vi "Format Basic String.vi"(10 "String":string) -> (2 "Formatted Basic String":string)   [LabVIEW 2019, in "BlueTOMLSerializer.lvlib"]
uses:
  BlueTOMLSerializer.lvlib
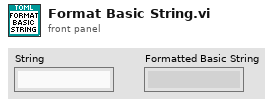
[diagram p1: front panel]
types:
  T1 = cluster{"replace string (\"\")":string, "replace string (\"\") 2":string}[]
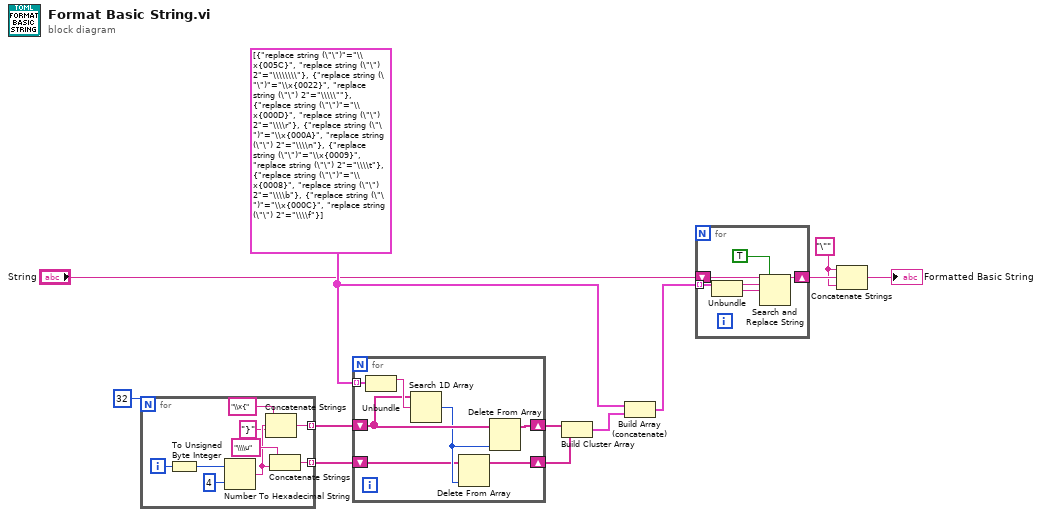
[diagram p0: block diagram]
diagram:
  w11 = "\"" ("string")
  w8 = T1 [{"replace string (\"\")"="\\x{005C}", "replace string (\"\") 2"="\\\\\\\\"}, {"replace string (\"\")"="\\x{0022}", "replace string (\"\") 2"="\\\\\""}, {"replace string (\"\")"="\\x{000D}", "replace string (\"\") 2"="\\\\r"}, {"replace string (\"\")"="\\x{000A}", "replace string (\"\") 2"="\\\\n"}, {"replace string (\"\")"="\\x{0009}", "replace string (\"\") 2"="\\\\t"}, {"replace string (\"\")"="\\x{0008}", "replace string (\"\") 2"="\\\\b"}, {"replace string (\"\")"="\\x{000C}", "replace string (\"\") 2"="\\\\f"}]
  n1 = for {
    N: 32 -> [_]
    tunnel: [w18] -> w5 mode=indexing
    tunnel: [w13] -> w4 mode=indexing
    i -> [w21]
    n2 = To Unsigned Byte Integer(number=w21) -> (unsigned 8bit integer=w16:u8)
    n3 = Number To Hexadecimal String(1:i16 4 ("width (-)"), 2:w16) -> (0:w15:string)
    n4 = Concatenate Strings("\\x{" ("string"), w15, "}" ("string")) -> (w13:string)
    n5 = Concatenate Strings("\\\\u" ("string"), w15) -> (w18:string)
  }
  n6 = for {
    tunnel: w8 -> [w28] mode=indexing
    shift-right: [w26] -> w6
    shift-left: w4 -> [w25]
    shift-right: [w23] -> w3
    shift-left: w5 -> [w22]
    n7 = Unbundle(w28) -> ("replace string (\"\")"=w27:string)  [unwired: 1 out]
    n8 = Search 1D Array(1D array=w25, element=w27) -> (index of element=w24:i32)  [unwired: 1 in]
    n9 = Delete From Array(array=w22, index=w24) -> (array with subset deleted=w23:string[])  [unwired: 1 in, 1 out]
    n10 = Delete From Array(array=w25, index=w24) -> (array with subset deleted=w26:string[])  [unwired: 1 in, 1 out]
  }
  n11 = Build Cluster Array(w6, w3) -> (w9:cluster{string, string}[])
  n12 = Build Array (concatenate)(w8, w9) -> (w7:T1)
  n13 = for {
    tunnel: w7 -> [w32] mode=indexing
    shift-right: [w29] -> w12
    shift-left: "String" -> [w34]
    n14 = Unbundle(w32) -> ("replace string (\"\")"=w31:string, "replace string (\"\") 2"=w30:string)
    n15 = Search and Replace String(replace all?=TRUE ("replace all? (F)"), input string=w34, search string=w31, replace string=w30) -> (result string=w29:string)  [unwired: 4 in, 3 out]
  }
  n16 = Concatenate Strings(w11, w12, w11) -> (→"Formatted Basic String":string)
